vi "Clear Single Error.vi"(8 "Error In":errorcluster, 11 "Error to clear":errorcluster) -> (0 "Error Out":errorcluster, 3 "specific error cleared?":bool)   [LabVIEW 2019]
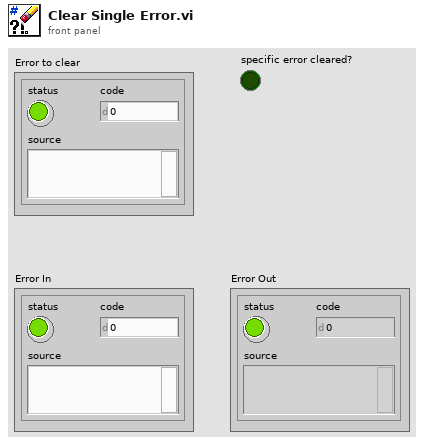
[diagram p1: front panel]
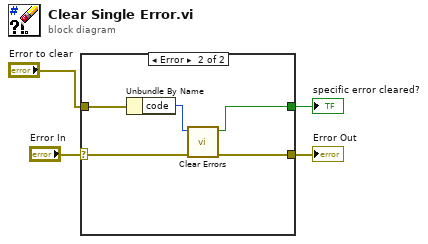
[diagram p0: block diagram]
diagram:
  n1 = case shown="Error" "Error In" {
    selector: "Error In" -> [w5 w8]
    tunnel: "Error to clear" -> [_ w10]
    tunnel: [w5 w9] -> w4
    tunnel: [_ w7] -> w2
    frame No Error {
    }
    frame Error {
      n2 = Unbundle By Name(w10) -> ("code"=w6:i32)
      n3 = call <vilib>:"Clear Errors.vi"("error in (no error)"=w8, "specific error code to clear (0: all)"=w6) -> ("error out"=w9:errorcluster, "specific error cleared?"=w7:bool)  [unwired: 4 in]
    }
  }
  "Error Out" <- w4
  "specific error cleared?" <- w2
